vi "Get Board Status.vi"(0 "Session Handle in":T1, 11 "error in (no error)":errorcluster) -> (4 "Session Handle out":T1, 6 "Ready?":bool, 15 "error out":errorcluster)   [LabVIEW 2015, in "Gas.lvclass"]
uses:
  Gas.lvclass
  Typedefs/Session Handle.ctl
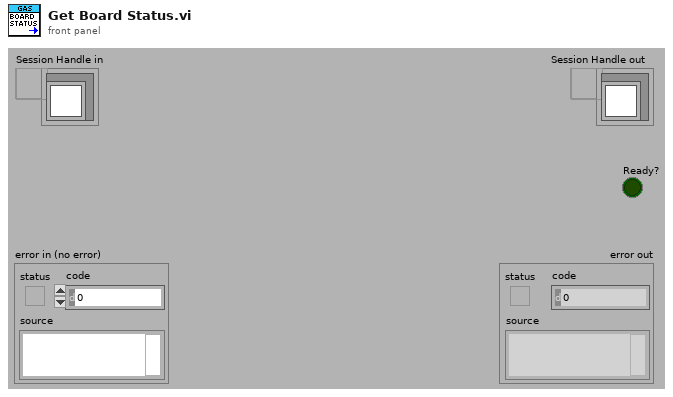
[diagram p1: front panel]
types:
  T1 = typedef "Gas.lvclass/Session Handle.ctl" = refnum<data-value>
  T2 = typedef "XNET Frame CAN.ctl" = cluster{"timestamp":timestamp, "payload":u8[], "identifier":u32, "type":T3, "extended?":bool, "echo?":bool}
  T3 = typedef "XNET Frame Type CAN.ctl" = u8
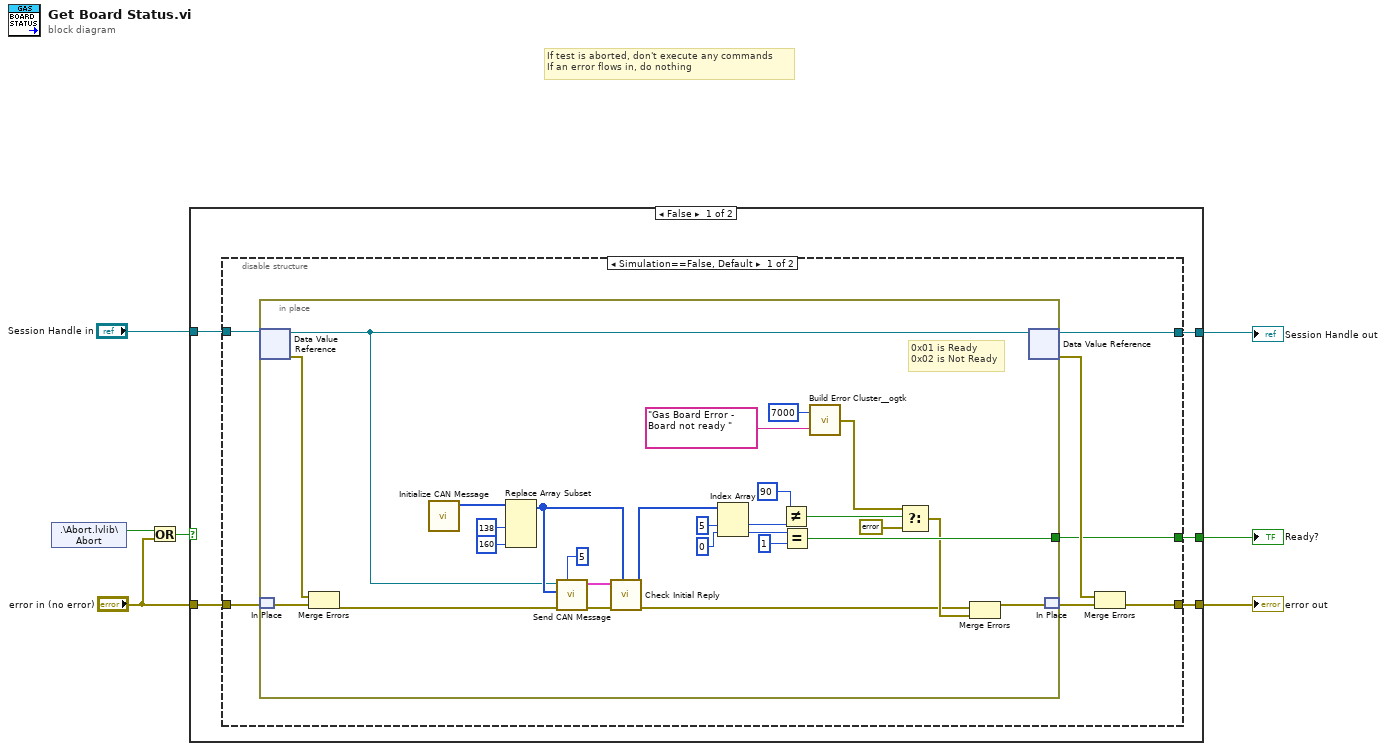
[diagram p0: block diagram]
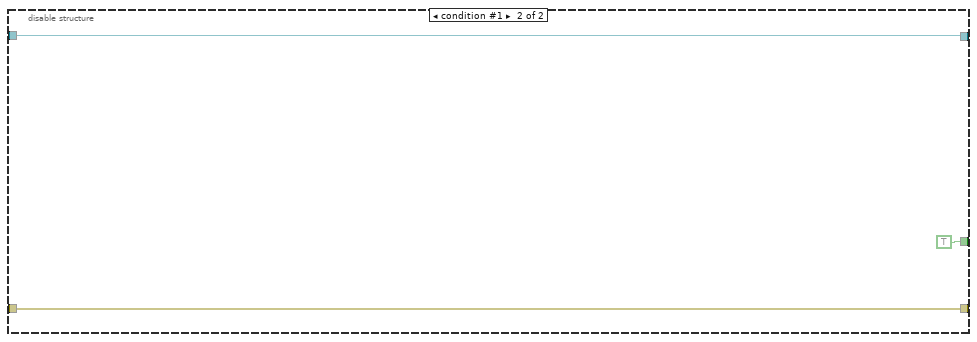
[diagram p2: hidden frame]
diagram:
  # "If test is aborted, don't execute any commands\nIf an error flows in, do nothing"
  n1 = shared-variable ".\\Abort.lvlib\\Abort"() -> (w4:bool)  [unwired: 1 in, 1 out]
  n2 = Or(x=w4, y="error in (no error)") -> (x .or. y?=w2:bool)
  n3 = case shown="False" w2 {
    tunnel: [w12 w51] -> w6
    tunnel: [w11 w50] -> w5
    tunnel: "Session Handle in" -> [w10 w51]
    tunnel: "error in (no error)" -> [w9 w50]
    tunnel: [w8 _] -> w1
    frame False {
      n4 = disable-structure shown="Simulation==False, Default" {
        disable-tunnel: [w19 w49] -> w12
        disable-tunnel: [w16 w48] -> w11
        disable-tunnel: w10 -> [w15 w49]
        disable-tunnel: w9 -> [w14 w48]
        disable-tunnel: [w13 TRUE] -> w8
        frame condition #0 (active) {
          n5 = in-place {
            in-place-border: [w23] -> w13
            # "0x01 is Ready\n0x02 is Not Ready"
            n6 = in-place-dvr #1(w15) -> (w37:refnum<class "Gas.lvclass">, w41:errorcluster)
            n7 = in-place-match #2(w14) -> (w40:errorcluster)
            n8 = Merge Errors(w41, w40) -> (w39:errorcluster)
            n9 = call "Initialize CAN Message.vi"() -> ("Initial Payload"=w43:u8[])  [unwired: 11 in]
            n10 = Replace Array Subset(array=w43, new element #1=u8 138 ("new element/subarray"), new element #2=u8 160 ("new element/subarray")) -> (w38:u8[])  [unwired: 2 in]
            n11 = call "Send CAN Message.vi"("Number of Retries"=5, "error in (no error)"=w39, "payload"=w38, "Gas In"=w37) -> ("error out"=w21:errorcluster, "Reply"=w35:T2[])  [unwired: 5 in, 1 out]
            n12 = call "Check Initial Reply.vi"("Write Message"=w38, "error in (no error)"=w21, "Reply"=w35) -> ("error out"=w20:errorcluster, "Data Packet"=w42:u8[])  [unwired: 5 in, 2 out]
            n13 = Index Array(array=w42, index #1=5 ("index"), index #2=0 ("index")) -> (element #1=w27:u8, element #2=w25:u8)
            n14 = Not Equal?(x=u8 90 ("new element/subarray"), y=w27) -> (x != y?=w30:bool)
            n15 = Equal?(x=w25, y=u8 1) -> (x = y?=w23:bool)
            n16 = call <userlib>:"Build Error Cluster__ogtk.vi"("String to Prepend to source (\"\")"="Gas Board Error - Board not ready " ("string"), "code"=7000) -> ("error out"=w32:errorcluster)
            n17 = Select(t=w32, s=w30, f=errorcluster {"status"=FALSE, "code"=0, "source"=""}) -> (s? t:f=w22:errorcluster)
            n18 = Merge Errors(w20, w22) -> (w44:errorcluster)
            n19 = in-place-dvr #1(w37) -> (w19:T1, w17:errorcluster)
            n20 = in-place-match #2(w44) -> (w18:errorcluster)
          }
          n21 = Merge Errors(w17, w18) -> (w16:errorcluster)
        }
        frame condition #1 {
        }
      }
    }
    frame True {
    }
  }
  "Session Handle out" <- w6
  "error out" <- w5
  "Ready?" <- w1
